vi "TestExec.Result, Set Mode.vi"(7 "Module Q Name":string, 8 "error in":errorcluster, 10 "Mode":string, 11 "Q In":refnum<queue>) -> (0 "error out":errorcluster, 3 "Q Out":refnum<queue>)   [LabVIEW 2019]
uses:
  <vilib>/KATE/Queues/Q.Element.ctl
  <vilib>/KATE/Queues/Queue Utils.lvlib
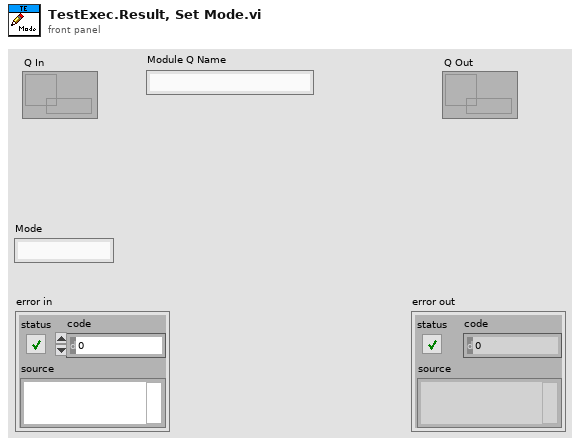
[diagram p1: front panel]
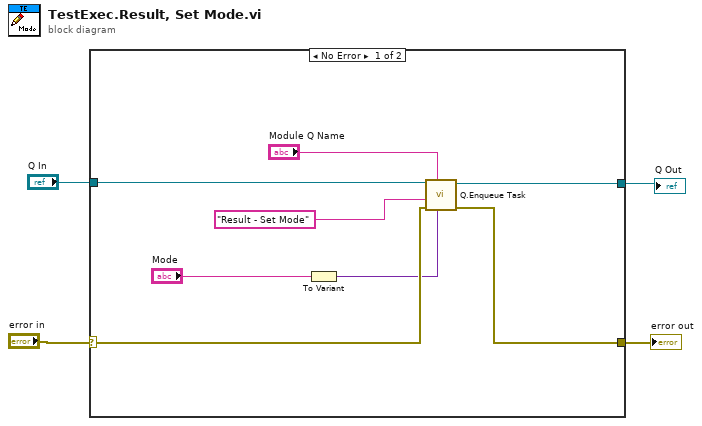
[diagram p0: block diagram]
diagram:
  n1 = case shown="No Error" "error in" {
    selector: "error in" -> [w10 w14]
    tunnel: [w11 w14] -> w3
    tunnel: [w6 w13] -> w2
    tunnel: "Q In" -> [w5 w13]
    frame No Error {
      n2 = To Variant(anything="Mode") -> (Variant=w8:variant)
      n3 = call <vilib>:"Q.Enqueue Task.vi"("Data1"=w8, "Q Name"="Module Q Name", "Error In"=w10, "Task Name"="Result - Set Mode" ("Cmd"), "Q In"=w5) -> ("error out"=w11:errorcluster, "Q Out"=w6:refnum<queue>)  [unwired: 5 in]
    }
    frame Error {
    }
  }
  "error out" <- w3
  "Q Out" <- w2
